vi "GENERADOR_29_01.vi"() -> ()   [LabVIEW 2013]
panel:
  in  "ENCENDER":bool
  out "Rango3 151-220":bool
  out "Rango2 101-150":bool
  out "Rango1-100":bool
  out "Rango 151-220":dbl
  out "Rango 101-150":dbl
  out "Rango 1-100":dbl
  out "Velocidad":i32(knob) scale=0.0..220.0
  # "SE TIENE QUE CONTAR CUANTAS VECES LA VELOCIDAD SE GENERA EN CADA UNO DE LO \nRANGOS Y SE ENCIENDE EL LED QUE CORRESPONDE A CADA UNO DE LOS RANGOS.\nHACERLO HASTA APAGAR EL AUTO"
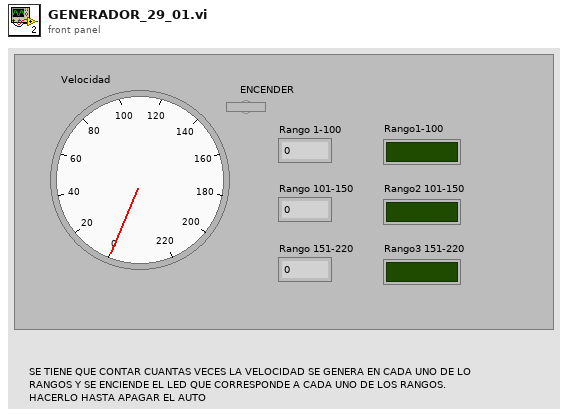
[diagram p1: front panel]
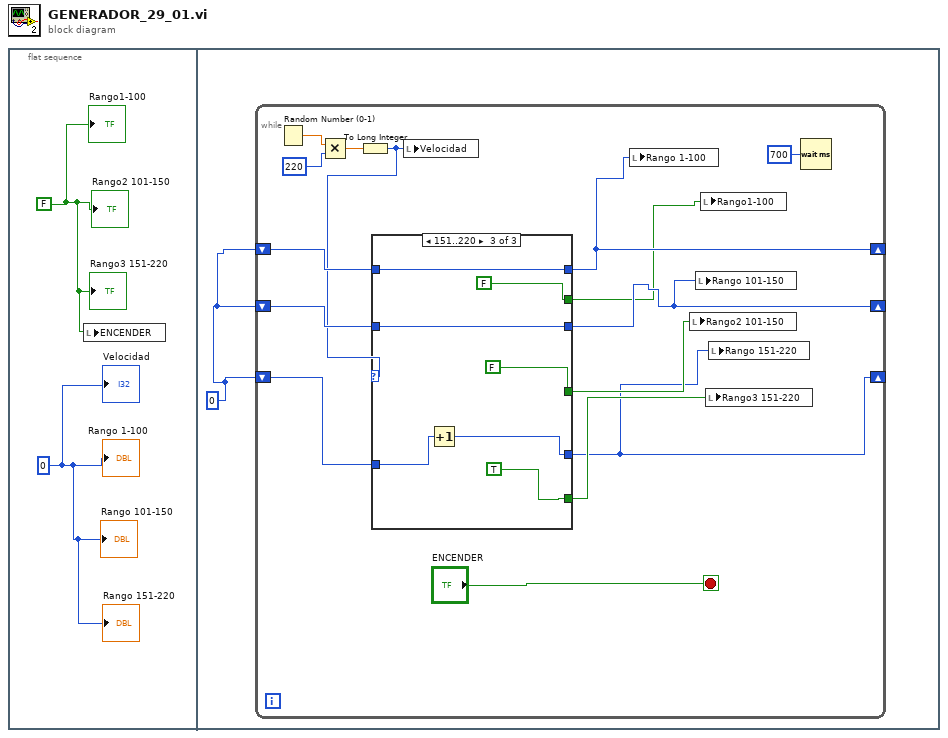
[diagram p0: block diagram]
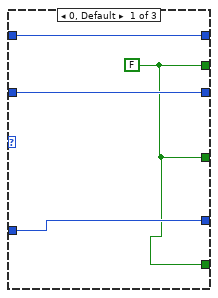
[diagram p2: hidden frame]
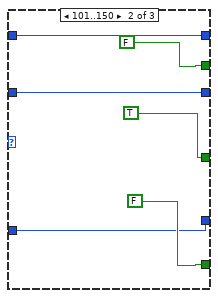
[diagram p3: hidden frame]
diagram:
  n1 = flat-sequence {
    frame #0 {
      w1 = FALSE
      w2 = 0
      n2 = local write "ENCENDER"(w1) -> ()
      "Velocidad" <- w2
      "Rango1-100" <- w1
      "Rango2 101-150" <- w1
      "Rango3 151-220" <- w1
      "Rango 1-100" <- w2
      "Rango 101-150" <- w2
      "Rango 151-220" <- w2
    }
    frame #1 {
      w3 = 0
      n3 = while {
        shift-right: [w13] -> _
        shift-left: w3 -> [w14]
        shift-right: [w11] -> _
        shift-left: w3 -> [w12]
        shift-right: [w6] -> _
        shift-left: w3 -> [w10]
        stop <- "ENCENDER" stop-if-true
        n4 = Random Number (0-1)() -> (number: 0 to 1=w17:dbl)
        n5 = Multiply(x=w17, y=220) -> (x*y=w15:dbl)
        n6 = To Long Integer(number=w15) -> (32bit integer=w4:i32)
        n7 = case shown="151..220" w4 {
          tunnel: w14 -> [w22 w25 w30]
          tunnel: [w22 w25 w30] -> w13
          tunnel: w12 -> [w21 w24 w29]
          tunnel: [w21 w24 w29] -> w11
          tunnel: [w20 w23 w31] -> w6
          tunnel: w10 -> [w20 w23 w32]
          tunnel: [w19 FALSE FALSE] -> w9
          tunnel: [w19 TRUE FALSE] -> w8
          tunnel: [w19 FALSE TRUE] -> w7
          frame 0, Default {
            w19 = FALSE
          }
          frame 101..150 {
          }
          frame 151..220 {
            n8 = Increment(x=w32) -> (x+1=w31:i32)
          }
        }
        n9 = local write "Velocidad"(w4) -> ()
        n10 = local write "Rango 1-100"(w13) -> ()
        n11 = local write "Rango2 101-150"(w8) -> ()
        n12 = local write "Rango 101-150"(w11) -> ()
        n13 = local write "Rango1-100"(w9) -> ()
        n14 = local write "Rango3 151-220"(w7) -> ()
        n15 = local write "Rango 151-220"(w6) -> ()
        n16 = Wait (ms)(milliseconds to wait=u32 700) -> ()  [unwired: 1 out]
      }
    }
  }
